vi "Write property.vi"(8 "error in (no error)":errorcluster, 10 "property":refnum<k21>, 11 "Relay in":refnum<class "Relay.lvclass">) -> (0 "error out":errorcluster, 3 "Relay out":refnum<class "Relay.lvclass">)   [LabVIEW 2015]
uses:
  Relay.lvclass
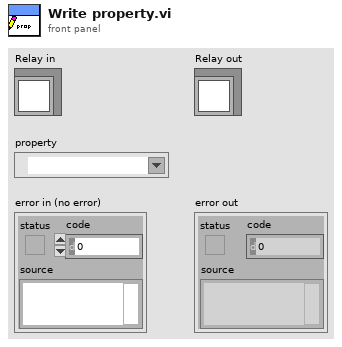
[diagram p1: front panel]
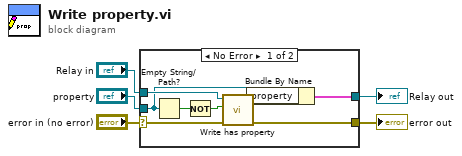
[diagram p0: block diagram]
diagram:
  n1 = case shown="No Error" "error in (no error)" {
    selector: "error in (no error)" -> [w7 w14]
    tunnel: [w6 w14] -> w4
    tunnel: [w13 w15] -> w2
    tunnel: "Relay in" -> [w12 w15]
    tunnel: "property" -> [w10 _]
    frame No Error {
      n2 = Empty String/Path?(string/path=w10) -> (empty?=w9:bool)
      n3 = Not(x=w9) -> (.not. x?=w8:bool)
      n4 = call "Write has property.vi"("error in (no error)"=w7, "has property"=w8, "Relay in"=w12) -> ("error out"=w6:errorcluster, "Relay out"=w11:refnum<class "Relay.lvclass">)  [unwired: 7 in]
      n5 = Bundle By Name(cluster=w11, "property"=w10) -> (w13:cluster{})
    }
    frame Error {
    }
  }
  "error out" <- w4
  "Relay out" <- w2
